vi "Subscriber.vi"() -> ()   [LabVIEW 2015]
uses:
  <vilib>/daq.io/MQTT LabVIEW Client/Controls/QoS.ctl
  <vilib>/daq.io/MQTT LabVIEW Client/Controls/DUP_Flag.ctl
  <vilib>/daq.io/MQTT LabVIEW Client/Controls/Retain_Flag.ctl
  <vilib>/daq.io/MQTT LabVIEW Client/Controls/Connect_Flags.ctl
  <vilib>/daq.io/MQTT LabVIEW Client/Controls/Connection_Return_Codes.ctl
  <vilib>/daq.io/MQTT LabVIEW Client/MQTT_Functions.lvlib
panel:
  in  "base path":path
  out "path":path
  out "concatenated string":string
  in  "Tab Control":enum32{"Session Controls", "Data"}(tab)
  in  "Connect Meta":T4={"QoS"=enum."At most once", "DUP"=FALSE, "Retain"=TRUE, "Keep Alive (sec)"=60}
  in  "Connect Flags":T5={"user name"=FALSE, "password"=FALSE, "will retain"=FALSE, "will flag"=FALSE, "clean session"=TRUE, "reserved"=FALSE, "will QoS"=enum."At most once"}
  in  "Subscriber ID":string="GETmyRIO"
  out "Subscriber Connection Status":T6=enum."Connection refused: not authorized"
  in  "Subscription Info Array":cluster{"Topic":string, "QoS":T1}[](array[cluster])=[{"Topic"="a/b", "QoS"=enum."At least once"}]
  out "Message":string="MQIsdp"
  in  "MQTT Broker":cluster{"address (IP)":string, "port":u16}={"address (IP)"="52.37.169.179", "port"=1883}
  in  "Stop":bool
  out "Samples Collected":i32
  in  "Sample Period(s)":dbl=1.0
  in  "?":bool=TRUE
  out "Data":dbl[][](array[numeric])
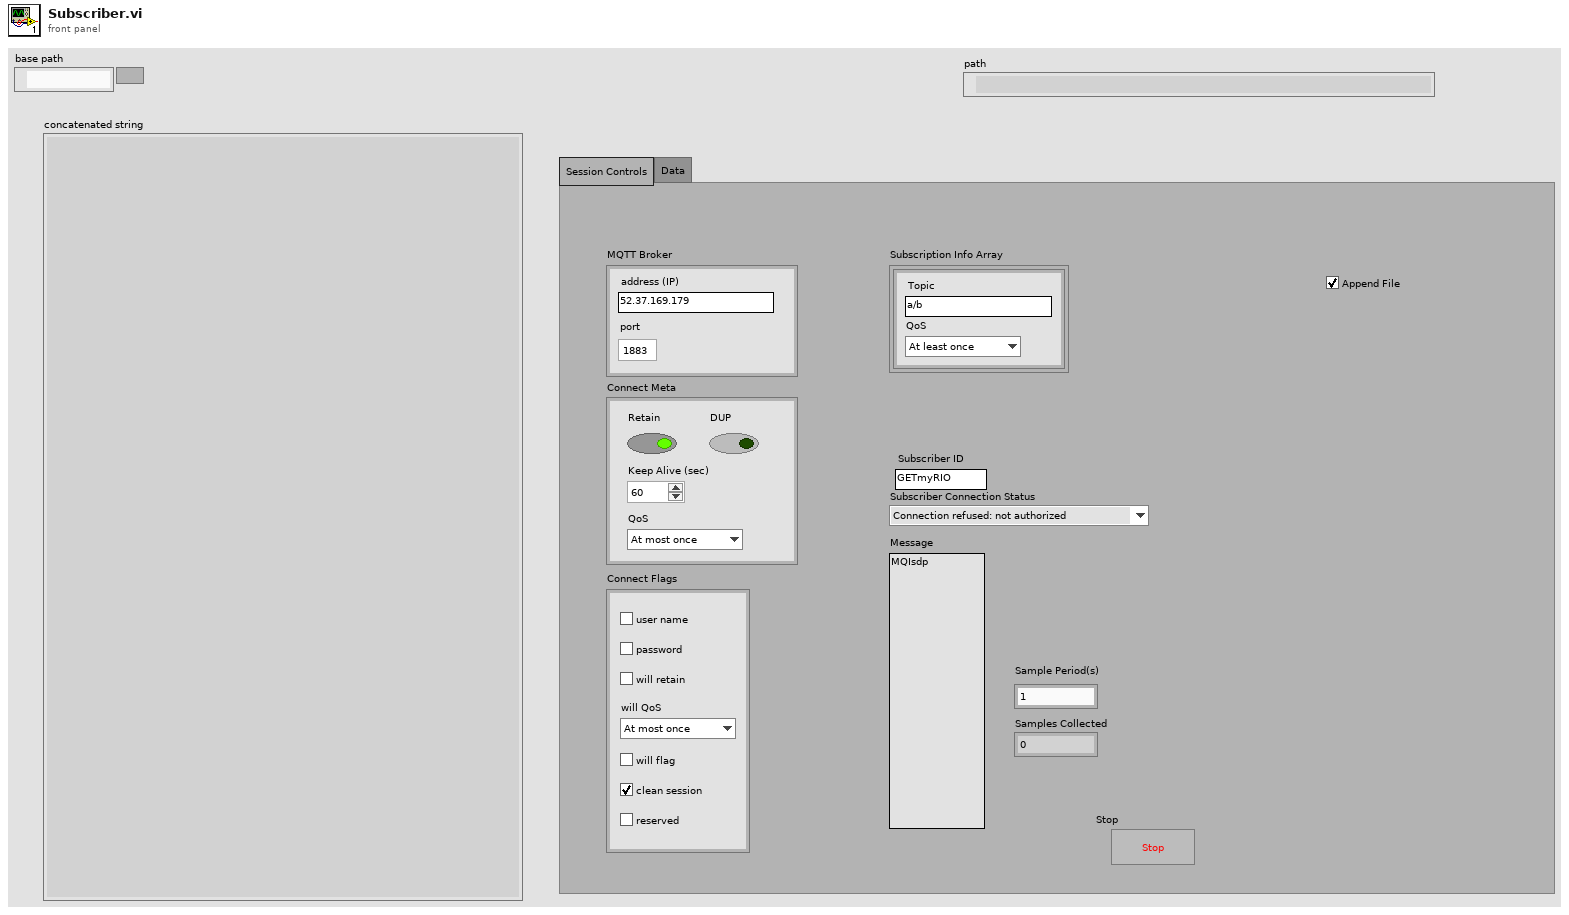
[diagram p1: front panel]
types:
  T1 = typedef "MQTT_Functions.lvlib/QoS.ctl" = enum8{"At most once", "At least once", "Exactly once", "Reserved"}
  T2 = typedef "MQTT_Functions.lvlib/DUP_Flag.ctl" = bool
  T3 = typedef "MQTT_Functions.lvlib/Retain_Flag.ctl" = bool
  T4 = cluster{"QoS":T1, "DUP":T2, "Retain":T3, "Keep Alive (sec)":u16}
  T5 = typedef "MQTT_Functions.lvlib/Connect_Flags.ctl" = cluster{"user name":bool, "password":bool, "will retain":bool, "will flag":bool, "clean session":bool, "reserved":bool, "will QoS":T1}
  T6 = typedef "MQTT_Functions.lvlib/Connection_Return_Codes.ctl" = enum16{"Connection accepted", "Connection refused: unacceptable protocol version", "Connection refused: identifier rejected", "Connection refused: Server unavailable", "Connection refused: bad user name or password", "Connection refused: not authorized"}
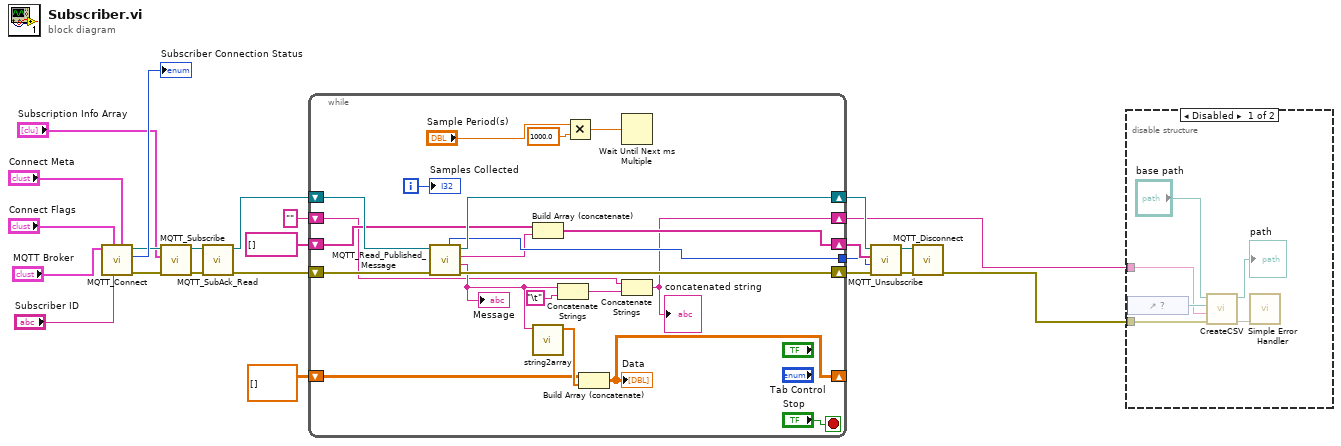
[diagram p0: block diagram]
diagram:
  n1 = call <vilib>:"MQTT_Connect.vi"("Connect Meta"="Connect Meta", "Client ID"="Subscriber ID", "Connect Flags"="Connect Flags", "MQTT Broker"="MQTT Broker") -> ("error out"=w15:errorcluster, "Connection Status"=→"Subscriber Connection Status":T6, "connection ID out"=w17:refnum<k5>)  [unwired: 5 in]
  n2 = call <vilib>:"MQTT_Subscribe.vi"("error in (no error)"=w15, "Subscription Info Array"="Subscription Info Array", "connection ID"=w17) -> ("error out"=w8:errorcluster, "connection ID out"=w9:refnum<k5>)  [unwired: 7 in]
  n3 = call <vilib>:"MQTT_SubAck_Read.vi"("error in (no error)"=w8, "connection ID"=w9) -> ("error out"=w7:errorcluster, "connection ID out"=w6:refnum<k5>)  [unwired: 7 in, 1 out]
  n4 = while {
    tunnel: [w41] -> w11
    shift-right: [w43] -> w16
    shift-left: w6 -> [w44]
    shift-right: [w30] -> w14
    shift-left: w7 -> [w32]
    shift-right: [w31] -> _
    shift-left: dbl[][] [] -> [w33]
    shift-right: [w42] -> w13
    shift-left: string[] [] -> [w34]
    shift-right: [w24] -> w1
    shift-left: "" -> [w26]
    i -> [w40]
    stop <- "Stop" stop-if-true
    n5 = call <vilib>:"MQTT_Read_Published_Message.vi"("error in (no error)"=w32, "connection ID"=w44) -> ("error out"=w30:errorcluster, "Message"=w27:string, "Topic Name"=w35:string, "connection ID out"=w43:refnum<k5>, "Message ID"=w41:u16)  [unwired: 4 in, 1 out]
    "Message" <- w27
    n6 = Build Array (concatenate)(w34, w35) -> (w42:string[])
    n7 = call "string2array.vi"("String"=w27) -> ("array"=w36:dbl[])  [unwired: 10 in]
    n8 = Concatenate Strings(w27, "\t") -> (w25:string)
    n9 = Multiply(x="Sample Period(s)", y=1000.0 ("milliseconds to wait")) -> (x*y=w39:dbl)
    n10 = Build Array (concatenate)(w33, w36) -> (w31:dbl[][])
    "Data" <- w31
    n11 = Wait Until Next ms Multiple(millisecond multiple=w39) -> ()  [unwired: 1 out]
    n12 = Concatenate Strings(w26, w25) -> (w24:string)
    "concatenated string" <- w24
    "Samples Collected" <- w40
  }
  n13 = call <vilib>:"MQTT_Unsubscribe.vi"("error in (no error)"=w14, "Message ID"=w11, "UnSubscribe Topic Array"=w13, "connection ID"=w16) -> ("error out"=w23:errorcluster, "connection ID out"=w22:refnum<k5>)  [unwired: 5 in, 1 out]
  n14 = call <vilib>:"MQTT_Disconnect.vi"("error in (no error)"=w23, "connection ID"=w22) -> ("error out"=w3:errorcluster)  [unwired: 9 in]
  n15 = disable-structure shown="Disabled" {
    disable-tunnel: w3 -> [w49 _]
    disable-tunnel: w1 -> [w45 _]
    frame Disabled {
      n16 = control-ref of="?"() -> (w48:refnum<vi>)
      n17 = call "CreateCSV.vi"(8:w49, "Data"=w45, "Append File?"=w48, "base path"="base path") -> (0:w50, "path"=→"path":path)  [unwired: 6 in]
      n18 = call <vilib>:"Simple Error Handler.vi"("error in (no error)"=w50) -> ()  [unwired: 4 in, 5 out]
    }
    frame Enabled {
    }
  }
